vi "hCalRT2013.vi"(0 "FPGA VI Reference In":refnum<k20>, 5 "cancelbutton":refnum<vi>, 7 "state":refnum<vi>, 9 "Acquired Samples":refnum<vi>, 11 "error in":errorcluster) -> (3 "Fehler":bool, 4 "FPGA VI Reference Out":refnum<k20>, 6 "Ref":i16[][](array[numeric]), 8 "Meas":i16[][](array[numeric]), 15 "error out":errorcluster)   [LabVIEW 2014]
uses:
  <vilib>/rvi/errors/niLvFpgaAdjustHostInterfaceError.vi
  <vilib>/Utility/error.llb/Error Cluster From Error Code.vi
  <vilib>/rvi/interface/nirviReadWriteControl/nirviReadWriteControl.xnode
  FPGA Bitfiles/W7XBolo2017_FPGATarget_FlorianDefault.lvbitx
  f_main_2014.vi
  NiFpgaLv.dll
panel:
  out "error in 2":errorcluster
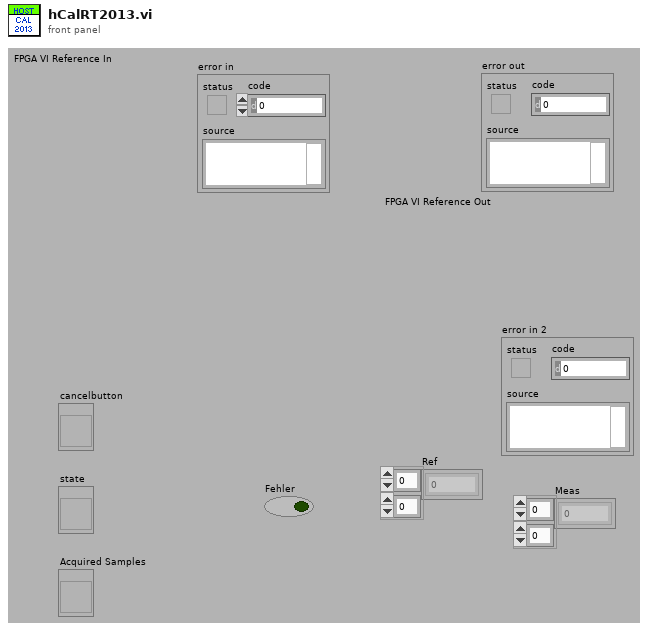
[diagram p1: front panel]
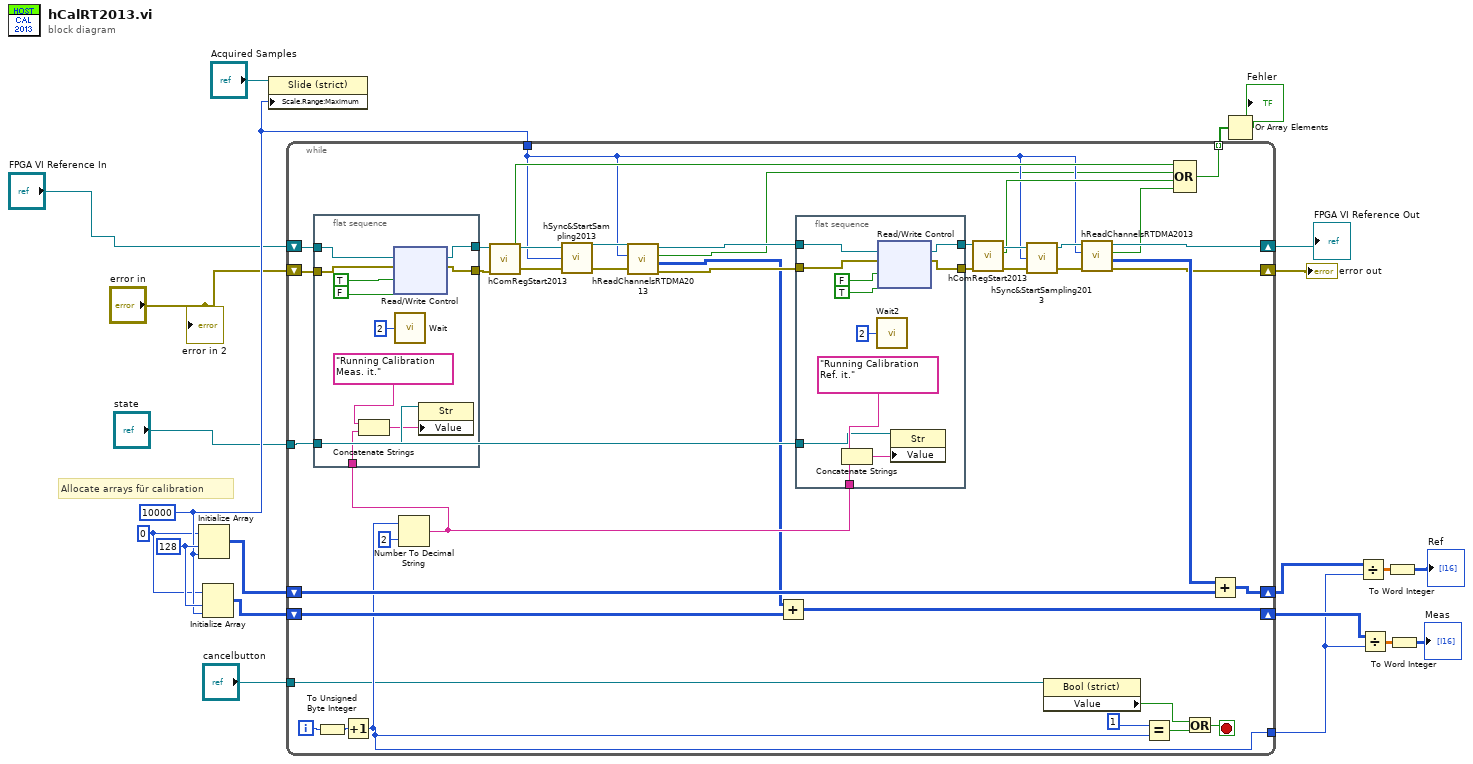
[diagram p0: block diagram]
diagram:
  w18 = 10000
  w19 = 128 ("dimension size")
  w15 = 0 ("element")
  # "Allocate arrays für calibration"
  n1 = Initialize Array(w15, w19, w18) -> (w17:i32[][])
  n2 = Initialize Array(w15, w19, w18) -> (w16:i32[][])
  n3 = property on="Property Node" class="Slide (strict)"(reference="Acquired Samples", "Scale.Range:Maximum"=w18) -> ()  [unwired: 1 in, 2 out]
  n4 = while {
    shift-right: [w34] -> w2
    shift-left: "FPGA VI Reference In" -> [w59]
    shift-right: [w31] -> w13
    shift-left: "error in" -> [w58]
    tunnel: w18 -> [w25]
    shift-right: [w47] -> w7
    shift-left: w17 -> [w48]
    shift-right: [w46] -> w6
    shift-left: w16 -> [w49]
    tunnel: [w41] -> w5
    tunnel: [w38] -> w21 mode=indexing
    tunnel: "cancelbutton" -> [w37]
    tunnel: "state" -> [w36]
    i -> [w55]
    stop <- w54 stop-if-true
    n5 = flat-sequence {
      tunnel: [w81] -> w62
      tunnel: [w80] -> w22
      tunnel: w59 -> [w79]
      tunnel: w58 -> [w78]
      tunnel: w52 -> [w76]
      tunnel: w36 -> [w75]
      frame #0 {
        n6 = Concatenate Strings("Running Calibration Meas. it." ("state"), w76) -> (w74:string)
        n7 = xnode "Read/Write Control"("FPGA VI Reference In"=w79, "error in"=w78, "RLY1"=TRUE ("RESET"), "RLY2"=FALSE ("RESET")) -> ("FPGA VI Reference Out"=w80:refnum<k20>, "error out"=w81:errorcluster)
        n8 = call "Wait"("Count(mSec)"=u8 2 ("Count(uSec)")) -> ()  [unwired: 1 out]
        n9 = property class="Str"(reference=w75, "Value"=w74) -> ()  [unwired: 1 in, 2 out]
      }
    }
    n10 = To Unsigned Byte Integer(number=w55) -> (unsigned 8bit integer=w51:u8)
    n11 = Increment(x=w51) -> (x+1=w41:u8)
    n12 = Number To Decimal String(number=w41, width (-)=u8 2) -> (decimal integer string=w52:string)
    n13 = call "hComRegStart2013.vi"("error in"=w62, "FPGA VI Reference In"=w22) -> ("error out"=w44:errorcluster, "Timed Out"=w40:bool, "FPGA VI Reference Out"=w45:refnum<k20>)  [unwired: 3 in]
    n14 = call "hSync&StartSampling2013.vi"("error in"=w44, "#Samples"=w25, "FPGA VI Reference In"=w45) -> ("error out"=w28:errorcluster, "FPGA VI Reference Out"=w29:refnum<k20>)  [unwired: 1 in]
    n15 = call "hReadChannelsRTDMA2013.vi"("FPGA VI Reference In"=w29, "Nsamples"=w25, "error in"=w28) -> ("FPGA VI Reference Out"=w27:refnum<k20>, "Fehler"=w24:bool, "RawArray"=w23:i16[][], "error out"=w26:errorcluster)  [unwired: 2 in]
    n16 = Add(x=w23, y=w49) -> (x+y=w46:i32[][])
    n17 = flat-sequence {
      tunnel: w27 -> [w70]
      tunnel: w26 -> [w69]
      tunnel: [w68] -> w61
      tunnel: [w67] -> w60
      tunnel: w52 -> [w64]
      tunnel: w36 -> [w63]
      frame #0 {
        n18 = Concatenate Strings("Running Calibration Ref. it." ("state"), w64) -> (w66:string)
        n19 = call "Wait2"("Count(mSec)"=u16 2 ("Count(uSec)")) -> ()  [unwired: 1 out]
        n20 = xnode "Read/Write Control"("FPGA VI Reference In"=w70, "error in"=w69, "RLY1"=FALSE ("RESET"), "RLY2"=TRUE ("RESET")) -> ("FPGA VI Reference Out"=w68:refnum<k20>, "error out"=w67:errorcluster)
        n21 = property class="Str"(reference=w63, "Value"=w66) -> ()  [unwired: 1 in, 2 out]
      }
    }
    n22 = call "hComRegStart2013.vi"("error in"=w60, "FPGA VI Reference In"=w61) -> ("error out"=w42:errorcluster, "Timed Out"=w39:bool, "FPGA VI Reference Out"=w43:refnum<k20>)  [unwired: 3 in]
    n23 = call "hSync&StartSampling2013.vi"("error in"=w42, "#Samples"=w25, "FPGA VI Reference In"=w43) -> ("error out"=w30:errorcluster, "FPGA VI Reference Out"=w35:refnum<k20>)  [unwired: 1 in]
    n24 = property class="Bool (strict)"(reference=w37) -> ("Value"=w50:bool)  [unwired: 1 in, 2 out]
    n25 = call "hReadChannelsRTDMA2013.vi"("FPGA VI Reference In"=w35, "Nsamples"=w25, "error in"=w30) -> ("FPGA VI Reference Out"=w34:refnum<k20>, "Fehler"=w32:bool, "RawArray"=w33:i16[][], "error out"=w31:errorcluster)  [unwired: 2 in]
    n26 = Equal?(x=u8 1, y=w41) -> (x = y?=w53:bool)
    n27 = Compound Arithmetic op=OR(w40, w24, w39, w32) -> (w38:bool)
    n28 = Or(x=w50, y=w53) -> (x .or. y?=w54:bool)
    n29 = Add(x=w33, y=w48) -> (x+y=w47:i32[][])
  }
  "error out" <- w13
  "FPGA VI Reference Out" <- w2
  n30 = Or Array Elements(Boolean array=w21) -> (logical OR=→"Fehler":bool)
  n31 = Divide(x=w7, y=w5) -> (x/y=w8:dbl[][])
  n32 = Divide(x=w6, y=w5) -> (x/y=w9:dbl[][])
  n33 = To Word Integer(number=w8) -> (16bit integer=→"Ref":i16[][])
  n34 = To Word Integer(number=w9) -> (16bit integer=→"Meas":i16[][])
  "error in 2" <- "error in"
